vi "Data Analog Output.vi"(0 "VISA resource name":refnum<visa-resource-name>, 7 "Analog Output (1)":dbl=1.0 min=1.0 max=2.0 step=1.0, 11 "error in (no error)":errorcluster) -> (4 "VISA resource name out":refnum<visa-resource-name>, 8 "Analog Output Read (%)":dbl min=-100.0 max=100.0 step=0.001 format="%.3f", 15 "error out":errorcluster)   [LabVIEW 2012, in "Lake Shore Cryotronics 218.lvlib"]
doc: "Displays the value of the selected analog output in percentage. Only the model 218S includes the Analog Output feature."
uses:
  <instrlib>/Lake Shore Cryotronics 218/Lake Shore Cryotronics 218.lvlib
panel:
  # "%"
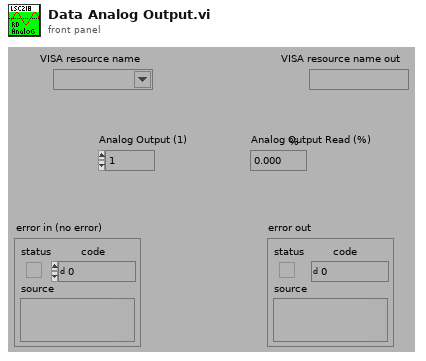
[diagram p1: front panel]
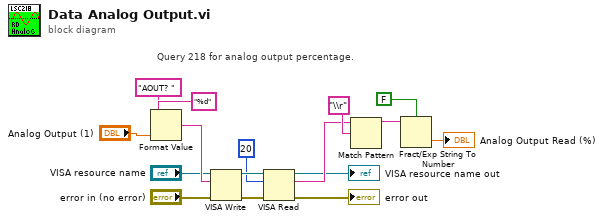
[diagram p0: block diagram]
diagram:
  # "Query 218 for analog output percentage."
  n1 = Format Value(string ("")="AOUT? ", format string="%d", value (0)="Analog Output (1)") -> (output string=w9:string)
  n2 = VISA Write(VISA resource name="VISA resource name", write buffer=w9, error in (no error)="error in (no error)") -> (VISA resource name out=w16:refnum<visa-resource-name>, error out=w15:errorcluster)  [unwired: 1 out]
  n3 = VISA Read(VISA resource name=w16, byte count=20, error in (no error)=w15) -> (VISA resource name out=→"VISA resource name out":refnum<visa-resource-name>, read buffer=w13:string, error out=→"error out":errorcluster)  [unwired: 1 out]
  n4 = Match Pattern(string=w13, regular expression="\\r") -> (before substring=w7:string)  [unwired: 1 in, 3 out]
  n5 = Fract/Exp String To Number(use system decimal point (T)=FALSE, string=w7) -> (number=→"Analog Output Read (%)":dbl)  [unwired: 2 in, 1 out]
